vi "qTGL.vi"(0 "System no.":i32=1 min=1 max=4 step=1, 2 "Trajectories to query":i32[](array[numeric]), 3 "All trajectories?":bool=TRUE, 5 "error in":errorcluster) -> (14 "Number of values":i32[](array[numeric]), 19 "error out":errorcluster)   [LabVIEW 2026]
doc: "Get number of values stored in trajectories. For further details, see Trajectories for Motion Paths in the controller user manual.\n\nC-867, C-884:"
panel:
  # "Get number of values stored in trajectories."
  # "Query"
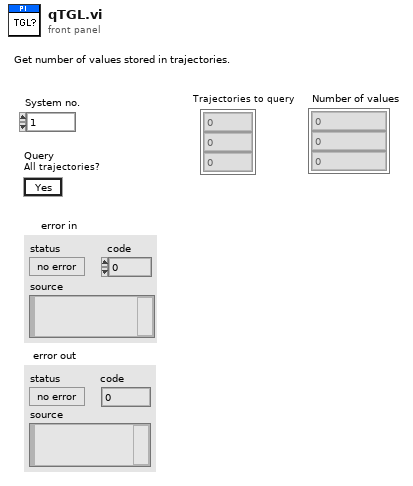
[diagram p1: front panel]
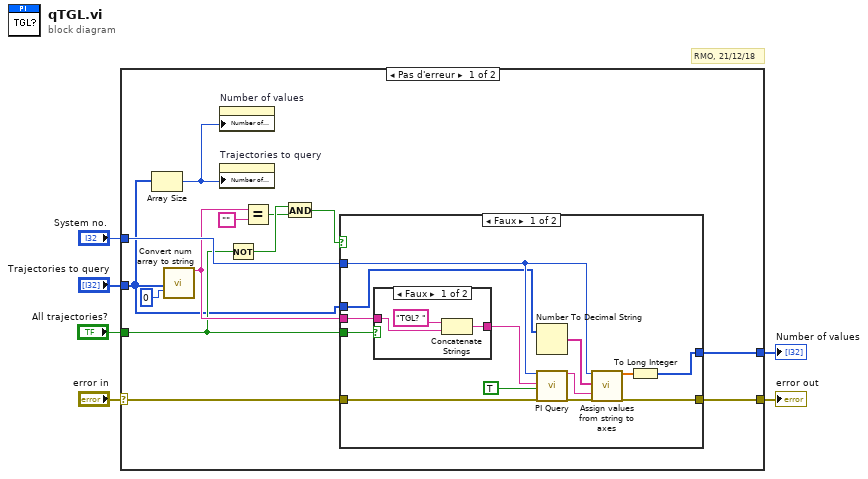
[diagram p0: block diagram]
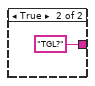
[diagram p2: hidden frame]
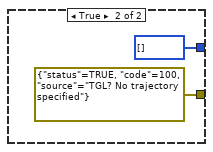
[diagram p3: hidden frame]
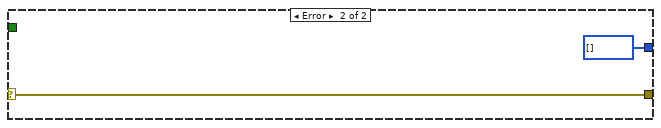
[diagram p4: hidden frame]
diagram:
  # "RMO, 21/12/18"
  n1 = case shown="Pas d'erreur" "error in" {
    selector: "error in" -> [w7 w39]
    tunnel: "Trajectories to query" -> [w8 _]
    tunnel: [w16 w39] -> w5
    tunnel: "System no." -> [w18 _]
    tunnel: "All trajectories?" -> [w10 _]
    tunnel: [w9 i32[] []] -> w2
    frame No Error {
      n2 = Array Size(array=w8) -> (size(s)=w17:i32)
      n3 = call "Convert num array to string.vi"("Num. values"=w8, "No. of digits"=i16 0) -> ("Output string"=w11:string)  [unwired: 17 out]
      n4 = property on="Number of values" class="Tabl (strict)"("Number of Rows"=w17) -> ()  [unwired: 2 in, 2 out]
      n5 = property on="Trajectories to query" class="Tabl (strict)"("Number of Rows"=w17) -> ()  [unwired: 2 in, 2 out]
      n6 = Not(x=w10) -> (.not. x?=w14:bool)
      n7 = Equal?(x=w11, y="" ("x")) -> (x = y?=w13:bool)
      n8 = And(x=w14, y=w13) -> (x .and. y?=w12:bool)
      n9 = case shown="Faux" w12 {
        tunnel: w18 -> [w30 _]
        tunnel: [w29 errorcluster {"status"=TRUE, "code"=100, "source"="TGL? No trajectory specified"} ("error out")] -> w16
        tunnel: w11 -> [w27 _]
        tunnel: w7 -> [w26 _]
        tunnel: w10 -> [w25 _]
        tunnel: [w24 i32[] []] -> w9
        tunnel: w8 -> [w23 _]
        frame False {
          n10 = case shown="Faux" w25 {
            tunnel: [w34 "TGL?"] -> w31
            tunnel: w27 -> [w33 _]
            frame False {
              n11 = Concatenate Strings("TGL? ", w33) -> (w34:string)
            }
            frame True {
            }
          }
          n12 = Number To Decimal String(number=w23) -> (decimal integer string=w22:string[])  [unwired: 1 out]
          n13 = call "PI Query.vi"("System no."=w30, "String to send"=w31, "Attach termination char.?"=TRUE ("Attach Linefeed?"), "error in"=w26) -> ("String read"=w20:string, "error out"=w21:errorcluster)  [unwired: 3 in, 11 out]
          n14 = call "Assign values from string to axes.vi"("System no."=w30, "Queried axes"=w22, "Input String"=w20, "error in"=w21) -> ("Values"=w28:dbl[], "error out"=w29:errorcluster)  [unwired: 5 in, 9 out]
          n15 = To Long Integer(number=w28) -> (32bit integer=w24:i32[])
        }
        frame True {
        }
      }
    }
    frame Error {
    }
  }
  "error out" <- w5
  "Number of values" <- w2
